vi "Read Devices armed.vi"(8 "error in (no error)":errorcluster, 11 "Application Controller in":refnum<class "Application Controller.lvclass">) -> (0 "error out":errorcluster, 2 "Devices armed":refnum<vi>, 3 "Application Controller out":refnum<class "Application Controller.lvclass">)   [LabVIEW 2019, in "Application Controller.lvclass"]
uses:
  Application Controller.lvclass
  Application Controller.lvclass/Application Controller.ctl
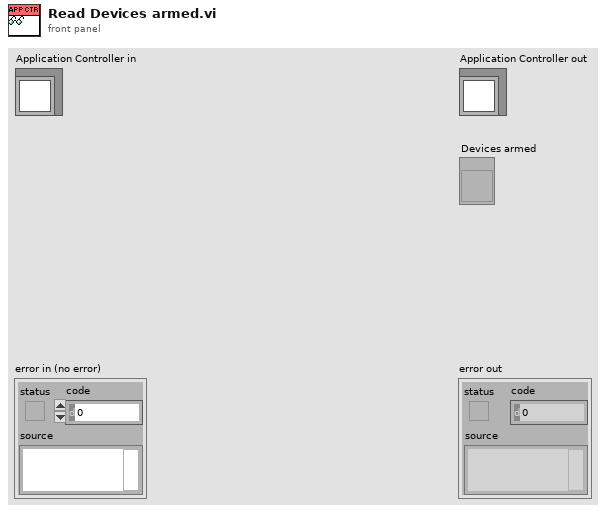
[diagram p1: front panel]
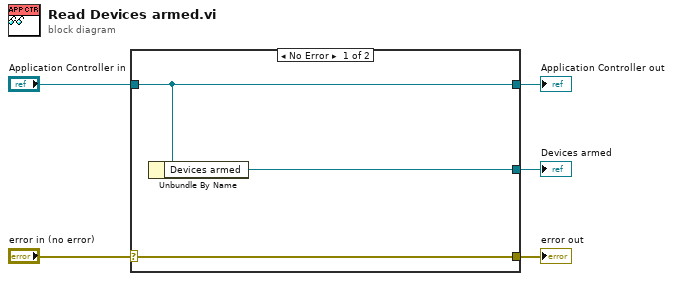
[diagram p0: block diagram]
diagram:
  n1 = case shown="No Error" "error in (no error)" {
    selector: "error in (no error)" -> [w8 w9]
    tunnel: [w8 w9] -> w4
    tunnel: [w7 w10] -> w2
    tunnel: "Application Controller in" -> [w7 w10]
    tunnel: [w6 _] -> w1
    frame No Error {
      n2 = Unbundle By Name(w7) -> ("Devices armed"=w6:refnum<vi>)
    }
    frame Error {
    }
  }
  "error out" <- w4
  "Application Controller out" <- w2
  "Devices armed" <- w1
